vi "ENCPID.vi"() -> ()   [LabVIEW 2019]
uses:
  <vilib>/addons/control/pid/pid.llb/PID (DBL).vi
  <vilib>/addons/control/pid/NI_PID_pid.lvlib
panel:
  in  "stop":bool
  out "Waveform Chart":i32(graph)
  in  "PID":T1={"proportional gain (Kc)"=0.010000000000000004, "integral time (Ti, min)"=0.001, "derivative time (Td, min)"=0.0} {"derivative time (Td, min)" format="%.4f"; "integral time (Ti, min)" format="%.3f"; "proportional gain (Kc)" format="%.2f"}
  out "Encoder":i32
  out "Error誤差":dbl
  in  "Target":dbl
  out "output":dbl format="%.2f"
  # "0.012"
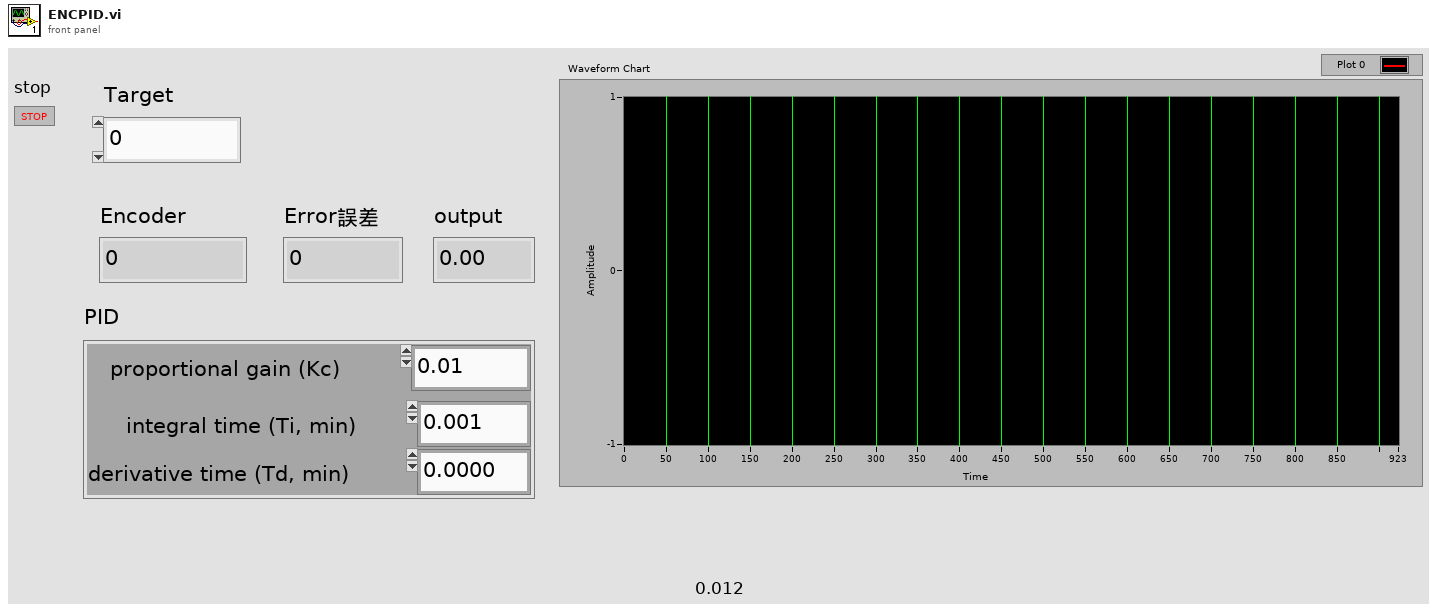
[diagram p1: front panel]
types:
  T1 = cluster{"proportional gain (Kc)":dbl, "integral time (Ti, min)":dbl, "derivative time (Td, min)":dbl}
  T2 = cluster{"ENC[0]":i32, "ENC[1]":i32, "ENC[2]":i32, "ENC[3]":i32}
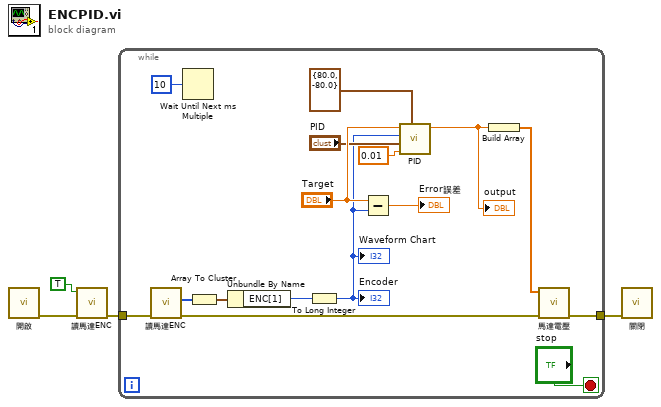
[diagram p0: block diagram]
diagram:
  n1 = call "開啟.vi"() -> ("Error/Flow Out"=w2:errorcluster)  [unwired: 11 in]
  n2 = call "讀馬達ENC.vi"("error in (no error)"=w2, "Reset"=TRUE ("Reset(F)")) -> ("error out"=w3:errorcluster)  [unwired: 8 in, 1 out]
  n3 = while {
    tunnel: w3 -> [w20]
    tunnel: [w16] -> w4
    stop <- "stop" stop-if-true
    n4 = call "讀馬達ENC.vi"("error in (no error)"=w20) -> ("error out"=w17:errorcluster, "ENC"=w19:i32[])  [unwired: 9 in]
    n5 = Wait Until Next ms Multiple(millisecond multiple=u32 10) -> ()  [unwired: 1 out]
    n6 = Array To Cluster(array=w19) -> (cluster=w18:T2)
    n7 = Unbundle By Name(w18) -> ("ENC[1]"=w6:i32)
    n8 = To Long Integer(number=w6) -> (32bit integer=w5:i32)
    "Encoder" <- w5
    "Waveform Chart" <- w5
    n9 = Subtract(x="Target", y=w5) -> (x-y=→"Error誤差":dbl)
    n10 = call-poly <vilib>:"PID.vi"("output range"=cluster{"output high":dbl, "output low":dbl} {"output high"=80.0, "output low"=-80.0}, "dt (s)"=0.01, "PID gains"="PID", "process variable"=w5, "setpoint"="Target") -> ("output"=w8:dbl)  [unwired: 5 in, 1 out]
    "output" <- w8
    n11 = Build Array(w8) -> (w11:dbl[])
    n12 = call "馬達電壓.vi"("error in (no error)"=w17, "DC_Pwr"=w11) -> ("error out"=w16:errorcluster)  [unwired: 9 in]
  }
  n13 = call "關閉.vi"("Error/Flow In"=w4) -> ()  [unwired: 11 in]
